vi "Configure Autozero.vi"(8 "error in (no error)":errorcluster, 9 "Autozero  (0: On)":u16(ring) items=["On", "Off"], 10 "Function (0: Volts)":u16(ring) items=["Volts", "Current", "Resistance"], 11 "VISA resource name":refnum<visa-resource-name>) -> (0 "error out":errorcluster, 3 "VISA resource name out":refnum<visa-resource-name>)   [LabVIEW 2025, in "Keithley 2450.lvlib"]
doc: "Enables or disables the autozero function on the instrument. Enabling autozero optimizes the instrument for accuracy, while disabling optimizes for speed."
uses:
  Keithley 2450.lvlib
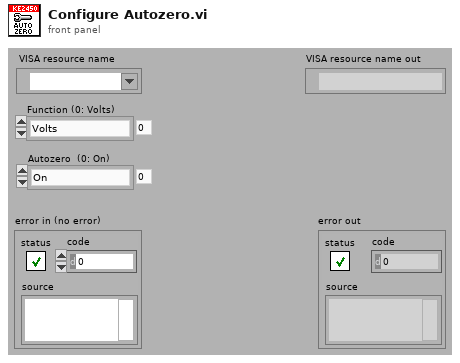
[diagram p1: front panel]
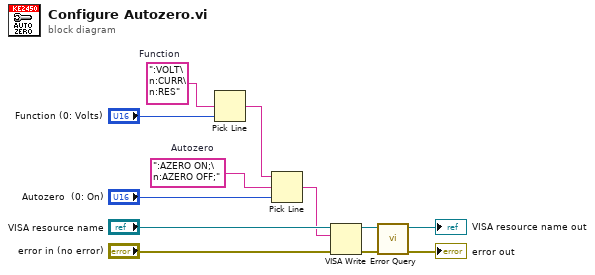
[diagram p0: block diagram]
diagram:
  w3 = ":VOLT\n:CURR\n:RES"  # Function
  w4 = ":AZERO ON;\n:AZERO OFF;"  # Autozero
  n1 = Pick Line(multi-line string=w3, line index="Function (0: Volts)") -> (output string=w1:string)  [unwired: 1 out]
  n2 = Pick Line(string ("")=w1, multi-line string=w4, line index="Autozero  (0: On)") -> (output string=w6:string)
  n3 = VISA Write(VISA resource name="VISA resource name", write buffer=w6, error in (no error)="error in (no error)") -> (VISA resource name out=w8:refnum<visa-resource-name>, error out=w7:errorcluster)  [unwired: 1 out]
  n4 = call "Error Query.vi"("error in (no error)"=w7, "VISA resource name"=w8) -> ("error out"=→"error out":errorcluster, "VISA resource name out"=→"VISA resource name out":refnum<visa-resource-name>)  [unwired: 8 out]
